vi "optionsAcq_offsetOpticalDetector.vi"(6 "ignore range violation (false)":bool, 8 "error in (no error)":errorcluster, 9 "readWrite":enum16{"read", "write"}(ring), 10 "detector offset":i32, 11 "Thorlabs_OSA200_64 in":refnum<class "OSA200.lvclass">) -> (0 "error out":errorcluster, 1 "status":string, 2 "offset read":i32, 3 "Thorlabs_OSA200_64 out":refnum<class "OSA200.lvclass">)   [LabVIEW 2010, in "OSA200.lvclass"]
uses:
  OSA200.lvclass
  OSA.lvclass
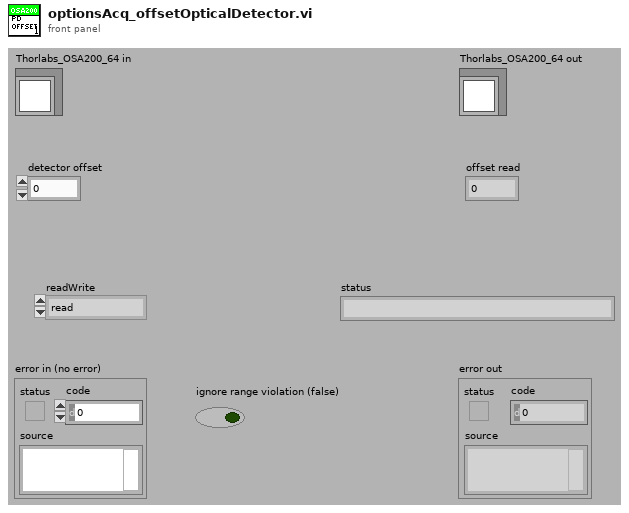
[diagram p1: front panel]
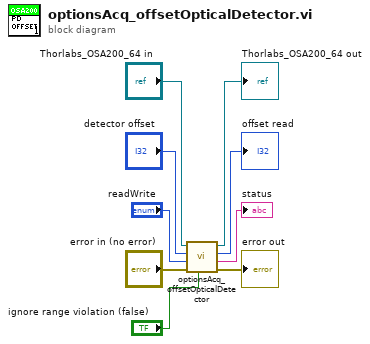
[diagram p0: block diagram]
diagram:
  n1 = call-parent "optionsAcq_offsetOpticalDetector.vi"("ignore range violation (false)"="ignore range violation (false)", "error in (no error)"="error in (no error)", "readWrite"="readWrite", "detector offset"="detector offset", "Thorlabs_OSA_64 in"="Thorlabs_OSA200_64 in") -> ("error out"=→"error out":errorcluster, "status"=→"status":string, "offset read"=→"offset read":i32, "Thorlabs_OSA_64 out"=→"Thorlabs_OSA200_64 out":refnum<class "OSA200.lvclass">)  [unwired: 3 in]
